vi "RFOVIs--GetVersion.vi"(8 "error in":errorcluster) -> (0 "error out":errorcluster, 3 "Version Info":T1={"Version"="4.0.0", "Build Number"=0, "Build Date/Time"=3400963200.0} {"Build Date/Time" format="%<%H:%M:%S\n%d/%m/%Y>T"})   [LabVIEW 2009]
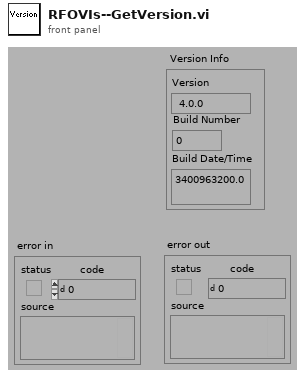
[diagram p1: front panel]
types:
  T1 = cluster{"Version":string, "Build Number":u32, "Build Date/Time":dbl}
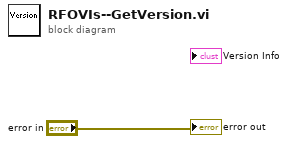
[diagram p0: block diagram]
diagram:
  "error out" <- "error in"
